vi "LHF.DB.Mongo.Collection.Update.Set.vi"(6 "Query":cluster{"Name":string, "JSON Value":string}, 8 "error in (no error)":errorcluster, 9 "Update":cluster{"Name":string, "JSON Value":string}, 10 "Collection":string, 11 "LHF.DB.Mongo in":refnum<class "LHF.DB.Mongo.lvclass">) -> (0 "error out":errorcluster, 3 "LHF.DB.Mongo out":refnum<class "LHF.DB.Mongo.lvclass">)   [LabVIEW 2013, in "LHF.DB.Mongo.lvclass"]
uses:
  LHF.DB.Mongo.lvclass
  C:/Users/schim/Desktop/Projetos/LabVIEW-MongoDB/src/Driver/MongoDB.Bson.dll
  Driver/MongoDB.Bson.dll
  C:/Users/schim/Desktop/Projetos/LabVIEW-MongoDB/src/Driver/MongoDB.Driver.dll
  Driver/MongoDB.Driver.dll
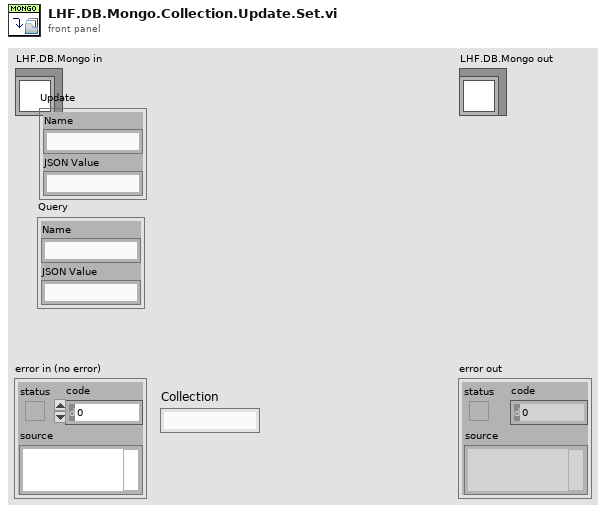
[diagram p1: front panel]
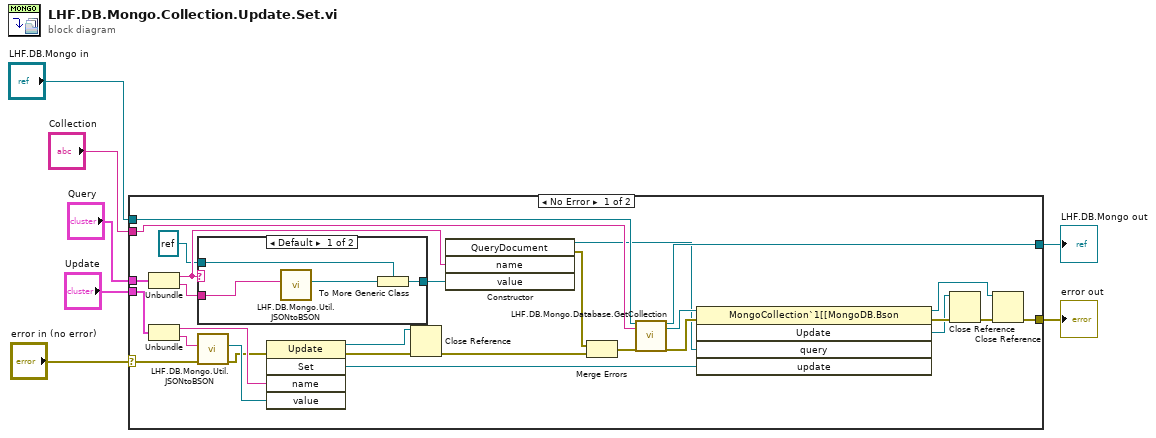
[diagram p0: block diagram]
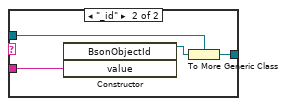
[diagram p2: hidden frame]
diagram:
  n1 = case shown="No Error" "error in (no error)" {
    selector: "error in (no error)" -> [w29 w45]
    tunnel: [w27 w45] -> w6
    tunnel: [w34 w44] -> w4
    tunnel: "LHF.DB.Mongo in" -> [w35 w44]
    tunnel: "Collection" -> [w33 _]
    tunnel: "Update" -> [w20 _]
    tunnel: "Query" -> [w21 _]
    frame No Error {
      n2 = Unbundle(w21) -> ("Name"=w18:string, "JSON Value"=w17:string)
      n3 = Unbundle(w20) -> ("Name"=w14:string, "JSON Value"=w19:string)
      n4 = case shown="Default" w18 {
        tunnel: [w37 w41] -> w16
        tunnel: w17 -> [w39 w43]
        tunnel: refnum<k24> refnum ("value") -> [w36 w40]
        frame Default {
          n5 = call "LHF.DB.Mongo.Util.JSONtoBSON.vi"("JSON data"=w39) -> ("BsonValue"=w38:refnum<k24>)  [unwired: 9 in, 1 out]
          n6 = To More Generic Class(target class=w36, reference=w38) -> (generic class reference=w37:refnum<k24>)
        }
        frame "_id" {
          n7 = constructor class="BsonObjectId"("value"=w43) -> (reference out=w42:refnum<k24>)  [unwired: 3 in, 3 out]
          n8 = To More Generic Class(target class=w40, reference=w42) -> (generic class reference=w41:refnum<k24>)
        }
      }
      n9 = call "LHF.DB.Mongo.Util.JSONtoBSON.vi"("error in (no error)"=w29, "JSON data"=w19) -> ("error out"=w11:errorcluster, "BsonValue"=w13:refnum<k24>)  [unwired: 8 in]
      n10 = invoke class="Update" method="Set"(error in=w11, "name"=w14, "value"=w13) -> (reference out=w10:refnum<k24>, error out=w9:errorcluster, "Set"=w12:refnum<k24>)  [unwired: 2 in, 2 out]
      n11 = Close Reference(reference=w10, error in (no error)=w9) -> (error out=w8:errorcluster)
      n12 = constructor class="QueryDocument"("name"=w18, "value"=w16) -> (reference out=w22:refnum<k24>, error out=w23:errorcluster)  [unwired: 3 in, 3 out]
      n13 = Merge Errors(w23, w8) -> (w31:errorcluster)
      n14 = call "LHF.DB.Mongo.Database.GetCollection.vi"("LHF.DB.Mongo in"=w35, "collectionName"=w33, "error in (no error)"=w31) -> ("LHF.DB.Mongo in"=w34:refnum<class "LHF.DB.Mongo.lvclass">, "MongoCollection"=w32:refnum<k24>, "error out"=w30:errorcluster)  [unwired: 14 in]
      n15 = invoke class="MongoCollection`1[[MongoDB.Bson" method="Update"(reference=w32, error in=w30, "query"=w22, "update"=w12) -> (reference out=w24:refnum<k24>, error out=w26:errorcluster, "Update"=w25:refnum<k24>)  [unwired: 1 in, 2 out]
      n16 = Close Reference(reference=w25, error in (no error)=w26) -> (error out=w28:errorcluster)
      n17 = Close Reference(reference=w24, error in (no error)=w28) -> (error out=w27:errorcluster)
    }
    frame Error {
    }
  }
  "error out" <- w6
  "LHF.DB.Mongo out" <- w4
